vi "1B_AnalyzeAmplitudeRamp_TimeOffset.vi"(1 "Measured":cluster{"X":dbl[], "Y":dbl[]}, 2 "Target":cluster{"X":dbl[], "Y":dbl[]}) -> (0 "delta x for the same Y ( time offset )":dbl)   [LabVIEW 2010]
uses:
  <vilib>/Analysis/NI_AALPro.lvlib
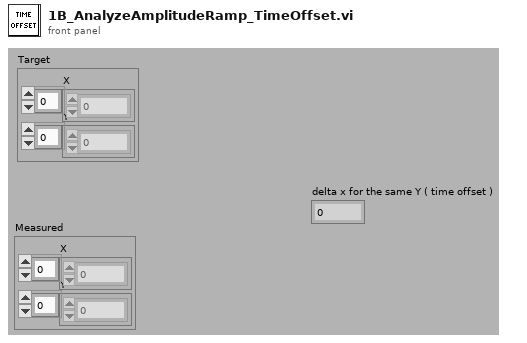
[diagram p1: front panel]
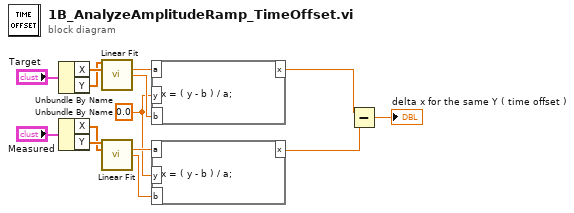
[diagram p0: block diagram]
diagram:
  w4 = 0.0 ("input variable")
  n1 = Unbundle By Name("Target") -> ("X"=w13:dbl[], "Y"=w12:dbl[])
  n2 = Unbundle By Name("Measured") -> ("X"=w10:dbl[], "Y"=w11:dbl[])
  n3 = call <vilib>:"Linear Fit.vi"("Y"=w12, "X"=w13) -> ("slope"=w6:dbl, "intercept"=w5:dbl)  [unwired: 9 in, 3 out]
  n4 = call <vilib>:"Linear Fit.vi"("Y"=w11, "X"=w10) -> ("slope"=w8:dbl, "intercept"=w7:dbl)  [unwired: 9 in, 3 out]
  n5 = formula code="x = ( y - b ) / a;"("a"=w6, "b"=w5, "y"=w4) -> ("x"=w3:dbl)
  n6 = formula code="x = ( y - b ) / a;"("a"=w8, "b"=w7, "y"=w4) -> ("x"=w2:dbl)
  n7 = Subtract(x=w3, y=w2) -> (x-y=→"delta x for the same Y ( time offset )":dbl)
